vi "test-merwe-scaled-sigma.vi"(8 "error in (no error)":errorcluster) -> (0 "error out":errorcluster, 3 "All Tests Passed":bool)   [LabVIEW 2019]
uses:
  <vilib>/Analysis/Matrix/Datatypes/RealMatrix.ctl
  <vilib>/Rock Robotics/WPI/ThirdParty/JAS_Junk/TrajLib/MERWE_SCALED_SIGMA_PTS.ctl
  <vilib>/Rock Robotics/WPI/ThirdParty/JAS_Junk/TrajLib/MatBuilder_Create.vi
  <vilib>/Rock Robotics/WPI/ThirdParty/JAS_Junk/TrajLib/MerweScSigPts_New.vi
  <vilib>/Rock Robotics/WPI/ThirdParty/JAS_Junk/TrajLib/Matrix_SetColumn.vi
  <vilib>/Rock Robotics/WPI/ThirdParty/JAS_Junk/TrajLib/Matrix_ExtractColumnVector.vi
  <vilib>/Rock Robotics/WPI/ThirdParty/JAS_Junk/TrajLib/Matrix_LltDecompose.vi
  <vilib>/Rock Robotics/WPI/ThirdParty/JAS_Junk/TrajLib/MatrixHelper_CoerceSize.vi
  <vilib>/Analysis/7linalg.llb/Cholesky Factorization.vi
  <vilib>/Analysis/7linalg.llb/Real Cholesky Factorization.vi
  <vilib>/Analysis/baseanly.llb/Full Cholesky Factorization.vi
  <vilib>/Analysis/baseanly.llb/Full Real Matrix Cholesky Factorization.vi
  <vilib>/Rock Robotics/WPI/ThirdParty/JAS_Junk/TrajLib/MerweScSigPts_ComputeWeights.vi
  <vilib>/Analysis/Matrix/Numeric/Multiply/Multiply.vi
  <vilib>/Analysis/Matrix/Numeric/Multiply/Multiply - RM,R.vi
  <vilib>/Analysis/Matrix/Numeric/Subtract/Subtract.vi
  <vilib>/Analysis/Matrix/Numeric/Subtract/Subtract - RM,RM.vi
  <vilib>/Analysis/Matrix/Numeric/Add/Add.vi
  <vilib>/Analysis/Matrix/Numeric/Add/Add - RM,RM.vi
  <vilib>/Rock Robotics/WPI/ThirdParty/JAS_Junk/TrajLib/Trajectory_Library.lvlib
  <vilib>/Analysis/Matrix/NI_Matrix.lvlib
panel:
  out "MerweScaledSigmaPts 1":T1
  out "Error 1":bool
  out "Passed 1":bool
  out "Equal 1":bool
  out "SigmaPoints  1":T2
  out "MerweScaledSigmaPts 0":T1
  out "Error 0":bool
  out "Passed 0":bool
  out "Equal 0":bool
  out "SigmaPoints  0":T2
  # "<?, 1>"
  # "<?, 1>"
  # "<?, 1>"
  # "<?, 1>"
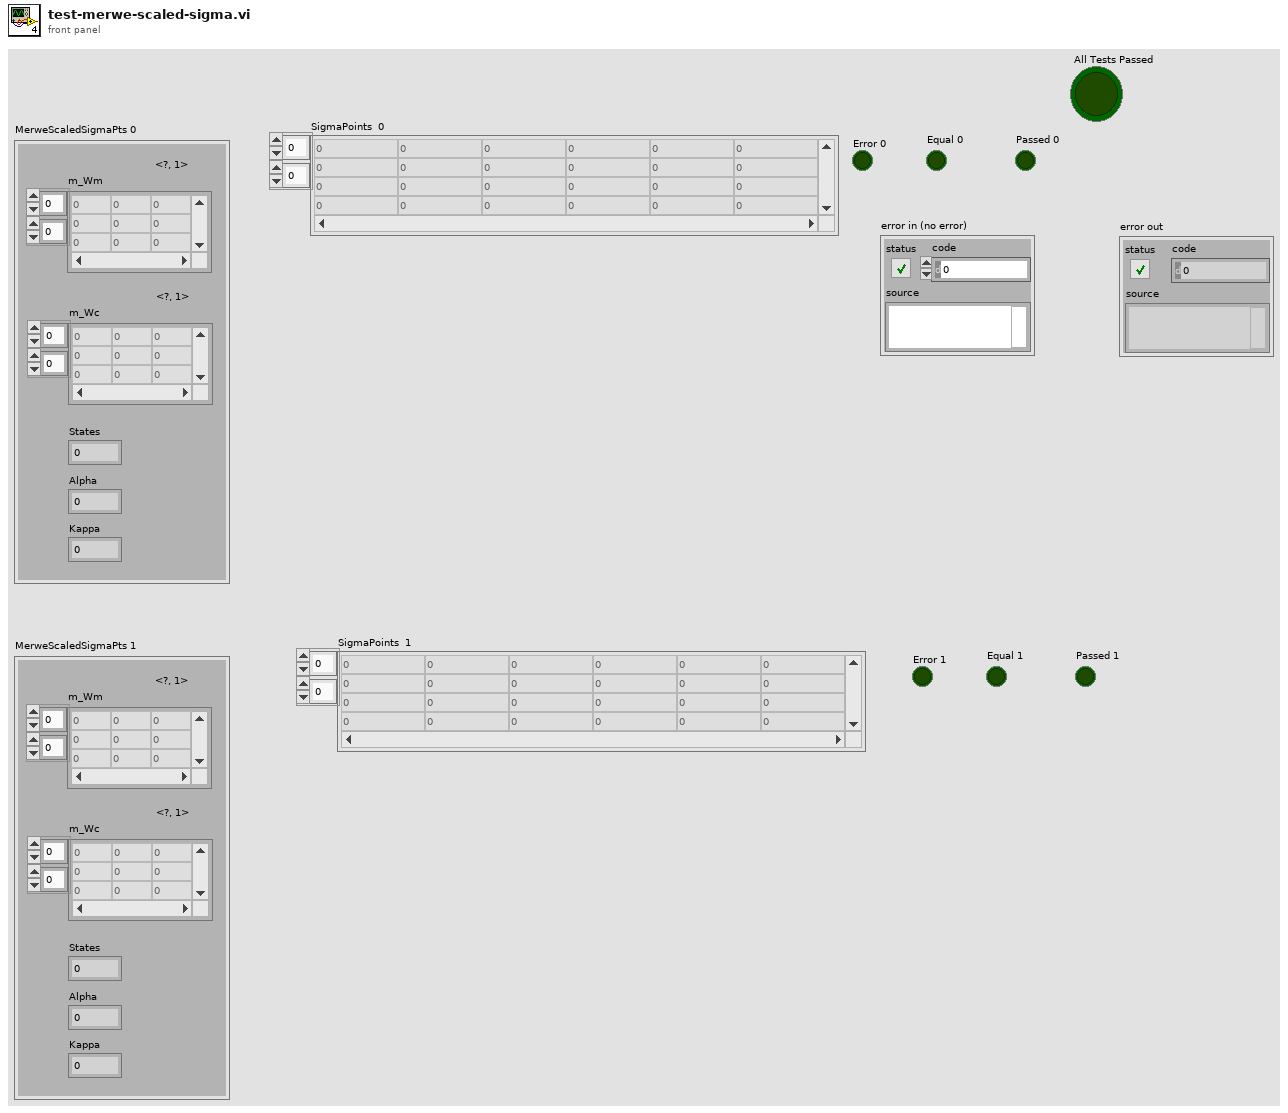
[diagram p1: front panel]
types:
  T1 = typedef "Trajectory_Library.lvlib/MERWE_SCALED_SIGMA_PTS.ctl" = cluster{"m_Wm":T2, "States":i32, "Alpha":dbl, "m_Wc":T2, "Kappa":i32}
  T2 = typedef "NI_Matrix.lvlib/RealMatrix.ctl" = dbl[][]
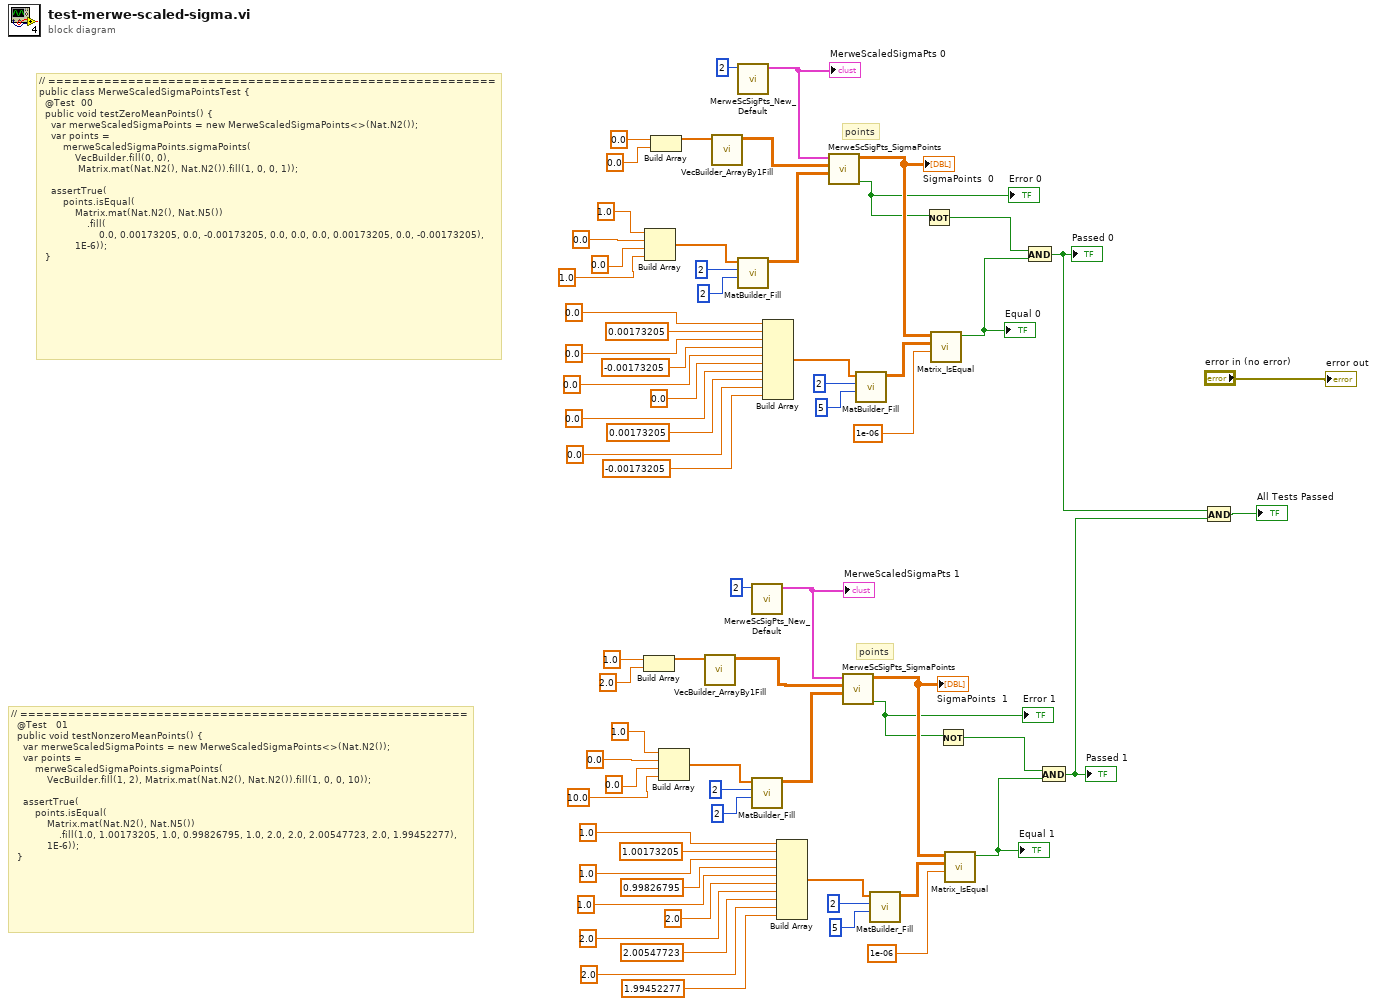
[diagram p0: block diagram]
diagram:
  # "points"
  # "points"
  # "// ========================================================\n  @Test   01\n  public void testNonzeroMeanPoints() {\n    var merweScaledSigmaPoints = new MerweScaledSigmaPoints<>(Nat.N2());\n    var points =\n        merweScaledSigmaPoints.sigmaPoints(\n            VecBuilder.fill(1, 2), Matrix.mat(Nat.N2(), Nat.N2()).fill(1, 0, 0, 10));\n\n    assertTrue(\n        points.isEqual(\n            Matrix.mat(Nat.N2(), Nat.N5())\n                .fill(1.0, 1.00173205, 1.0, 0.99826795, 1.0, 2.0, 2.0, 2.00547723, 2.0, 1.99452277),\n            1E-6));\n  }"
  # "// ========================================================\npublic class MerweScaledSigmaPointsTest {\n  @Test  00\n  public void testZeroMeanPoints() {\n    var merweScaledSigmaPoints = new MerweScaledSigmaPoints<>(Nat.N2());\n    var points =\n        merweScaledSigmaPoints.sigmaPoints(\n            VecBuilder.fill(0, 0), \n             Matrix.mat(Nat.N2(), Nat.N2()).fill(1, 0, 0, 1));\n\n    assertTrue(\n        points.isEqual(\n            Matrix.mat(Nat.N2(), Nat.N5())\n                .fill(\n                    0.0, 0.00173205, 0.0, -0.00173205, 0.0, 0.0, 0.0, 0.00173205, 0.0, -0.00173205),\n            1E-6));\n  }"
  n1 = Build Array(1.0 ("element"), 2.0 ("element")) -> (w7:dbl[])
  n2 = Build Array(1.0 ("element"), 0.0 ("element"), 0.0 ("element"), 1.0 ("element")) -> (w67:dbl[])
  n3 = Build Array(0.0 ("element"), 0.0 ("element")) -> (w11:dbl[])
  n4 = Build Array(1.0 ("element"), 0.0 ("element"), 0.0 ("element"), 10.0 ("element")) -> (w38:dbl[])
  n5 = call <vilib>:"VecBuilder_ArrayBy1Fill.vi"("R Array"=w7) -> ("Output Vector"=w5:T2)  [unwired: 10 in]
  n6 = call <vilib>:"VecBuilder_ArrayBy1Fill.vi"("R Array"=w11) -> ("Output Vector"=w9:T2)  [unwired: 10 in]
  n7 = call <vilib>:"MerweScSigPts_New_Default.vi"("States"=2) -> ("MerweScaledSigmaPts"=w69:T1)  [unwired: 10 in]
  "MerweScaledSigmaPts 0" <- w69
  n8 = call <vilib>:"MatBuilder_Fill.vi"("Columns"=2, "Rows"=2, "Value List"=w67) -> ("output matrix"=w60:T2)  [unwired: 8 in]
  n9 = call <vilib>:"MerweScSigPts_New_Default.vi"("States"=2) -> ("MerweScaledSigmaPts"=w39:T1)  [unwired: 10 in]
  "MerweScaledSigmaPts 1" <- w39
  n10 = call <vilib>:"MatBuilder_Fill.vi"("Columns"=2, "Rows"=2, "Value List"=w38) -> ("output matrix"=w31:T2)  [unwired: 8 in]
  n11 = Build Array(0.0 ("element"), 0.00173205 ("element"), 0.0 ("element"), -0.00173205 ("element"), 0.0 ("element"), 0.0 ("element"), 0.0 ("element"), 0.00173205 ("element"), 0.0 ("element"), -0.00173205 ("element")) -> (w59:dbl[])
  n12 = Build Array(1.0 ("element"), 1.00173205 ("element"), 1.0 ("element"), 0.99826795 ("element"), 1.0 ("element"), 2.0 ("element"), 2.0 ("element"), 2.00547723 ("element"), 2.0 ("element"), 1.99452277 ("element")) -> (w30:dbl[])
  n13 = call <vilib>:"MerweScSigPts_SigmaPoints.vi"("P"=w60, "X"=w9, "MerweScaledSigmaPts"=w69) -> ("Error"=w42:bool, "SigmaPoints"=w46:T2)  [unwired: 7 in]
  "SigmaPoints  0" <- w46
  "Error 0" <- w42
  n14 = call <vilib>:"MerweScSigPts_SigmaPoints.vi"("P"=w31, "X"=w5, "MerweScaledSigmaPts"=w39) -> ("Error"=w13:bool, "SigmaPoints"=w17:T2)  [unwired: 7 in]
  "SigmaPoints  1" <- w17
  "Error 1" <- w13
  n15 = call <vilib>:"MatBuilder_Fill.vi"("Columns"=5, "Rows"=2, "Value List"=w59) -> ("output matrix"=w45:T2)  [unwired: 8 in]
  n16 = call <vilib>:"MatBuilder_Fill.vi"("Columns"=5, "Rows"=2, "Value List"=w30) -> ("output matrix"=w16:T2)  [unwired: 8 in]
  n17 = Not(x=w42) -> (.not. x?=w43:bool)
  n18 = call <vilib>:"Matrix_IsEqual.vi"("Tolerance"=1e-06, "other"=w45, "input matrix"=w46) -> ("Equal"=w41:bool)  [unwired: 8 in]
  "Equal 0" <- w41
  n19 = Not(x=w13) -> (.not. x?=w14:bool)
  n20 = call <vilib>:"Matrix_IsEqual.vi"("Tolerance"=1e-06, "other"=w16, "input matrix"=w17) -> ("Equal"=w12:bool)  [unwired: 8 in]
  "Equal 1" <- w12
  n21 = And(x=w43, y=w41) -> (x .and. y?=w4:bool)
  "Passed 0" <- w4
  n22 = And(x=w14, y=w12) -> (x .and. y?=w2:bool)
  "Passed 1" <- w2
  n23 = And(x=w4, y=w2) -> (x .and. y?=→"All Tests Passed":bool)
  "error out" <- "error in (no error)"
